vi "DecodeMonitorHeader(FHW1).vi"(11 "fhw1":u32 format="%.0x") -> (3 "FHW1":T1)   [LabVIEW 2020, in "AIM664LV.lvlib"]
uses:
  AIM664LV.lvlib
  _controls/monitor_fhw1_type.ctl
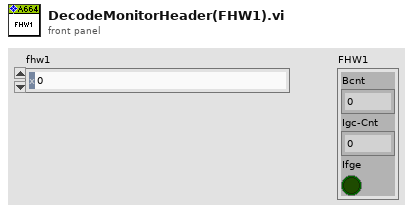
[diagram p1: front panel]
types:
  T1 = typedef "AIM664LV.lvlib/monitor_fhw1_type.ctl" = cluster{"Bcnt":u16, "Igc-Cnt":u16, "Ifge":bool}
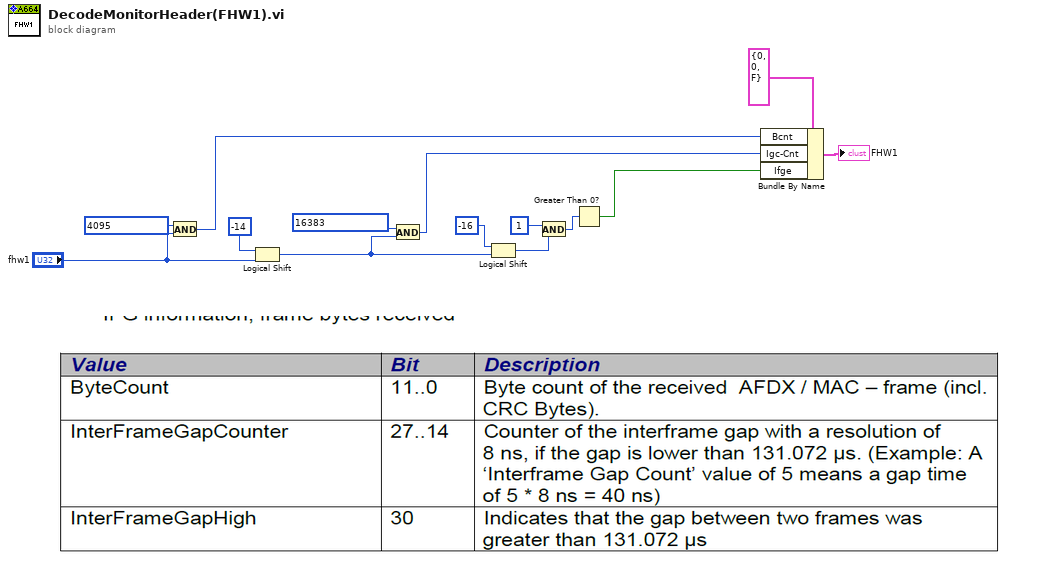
[diagram p0: block diagram]
diagram:
  n1 = And(x=u32 4095 ("Numeric"), y="fhw1") -> (x .and. y?=w11:u32)
  n2 = Logical Shift(y=i16 -14, x="fhw1") -> (x << y=w6:u32)
  n3 = And(x=u32 16383 ("Numeric"), y=w6) -> (x .and. y?=w7:u32)
  n4 = Logical Shift(y=i16 -16, x=w6) -> (x << y=w3:u32)
  n5 = And(x=u32 1 ("Numeric"), y=w3) -> (x .and. y?=w5:u32)
  n6 = Greater Than 0?(x=w5) -> (x > 0?=w4:bool)
  n7 = Bundle By Name(cluster=T1 {"Bcnt"=0, "Igc-Cnt"=0, "Ifge"=FALSE} ("FHW1"), "Bcnt"=w11, "Igc-Cnt"=w7, "Ifge"=w4) -> (→"FHW1":T1)
